vi "Update Width.vi"(8 "error in (no error)":errorcluster, 10 "Width":u16, 11 "ButtonControlEditorPanel in":refnum<class "ButtonControlEditorPanel.lvclass">) -> (0 "error out":errorcluster, 3 "ButtonControlEditorPanel out":refnum<class "ButtonControlEditorPanel.lvclass">)   [LabVIEW 2020, in "VolatusGUIControls.lvlib" / "ButtonControlEditorPanel.lvclass"]
uses:
  ButtonControlEditorPanel.lvclass
  ButtonControlEditorPanel.lvclass/ButtonControlEditorPanel.ctl
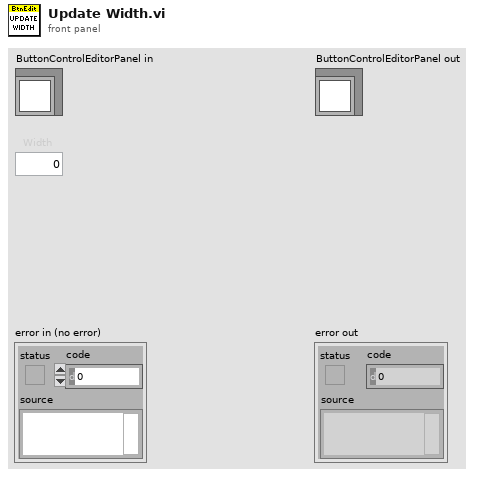
[diagram p1: front panel]
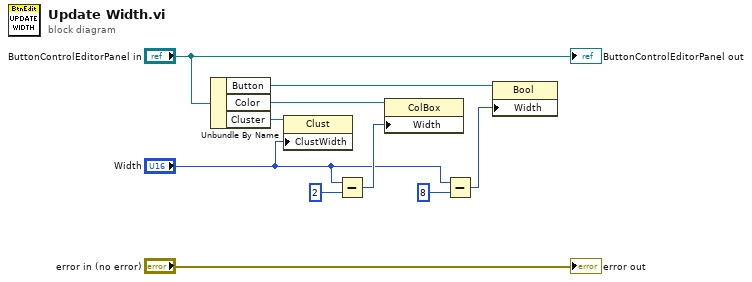
[diagram p0: block diagram]
diagram:
  n1 = Unbundle By Name("ButtonControlEditorPanel in") -> ("Button"=w8:refnum<vi>, "Color"=w7:refnum<vi>, "Cluster"=w6:refnum<vi>)
  n2 = property class="Clust"(reference=w6, "ClustWidth"="Width") -> ()  [unwired: 1 in, 2 out]
  n3 = Subtract(x="Width", y=u16 2) -> (x-y=w2:u16)
  n4 = property class="ColBox"(reference=w7, "Width"=w2) -> ()  [unwired: 1 in, 2 out]
  n5 = Subtract(x="Width", y=u16 8) -> (x-y=w4:u16)
  n6 = property class="Bool"(reference=w8, "Width"=w4) -> ()  [unwired: 1 in, 2 out]
  "error out" <- "error in (no error)"
  "ButtonControlEditorPanel out" <- "ButtonControlEditorPanel in"
